vi "meter_buffered - one channel.vi"(7 "Samples":dbl=50.0 format="%#_13g", 8 "error in":errorcluster, 9 "Channel":u16(ring) items=["PD 1", "PD 2", "PD 3"], 10 "PD Range":dbl=3e-05 format="%#_13g", 11 "meter-VISA":refnum<visa-resource-name>) -> (0 "error out":errorcluster, 1 "avg":dbl, 2 "ch data":dbl[](array[numeric]), 3 "meter-VISA-out":refnum<visa-resource-name>, 4 "stdev":dbl)   [LabVIEW 2024]
uses:
  <instrlib>/Keithley 6517/Keithley 6517.lvlib
  <vilib>/Analysis/NI_AALBase.lvlib
panel:
  out "read buffer":string
  out "vi_runtime":u32
  out "pd1_size":i32
  out "pd1_data":dbl[](array[numeric])
  out "cmd":string
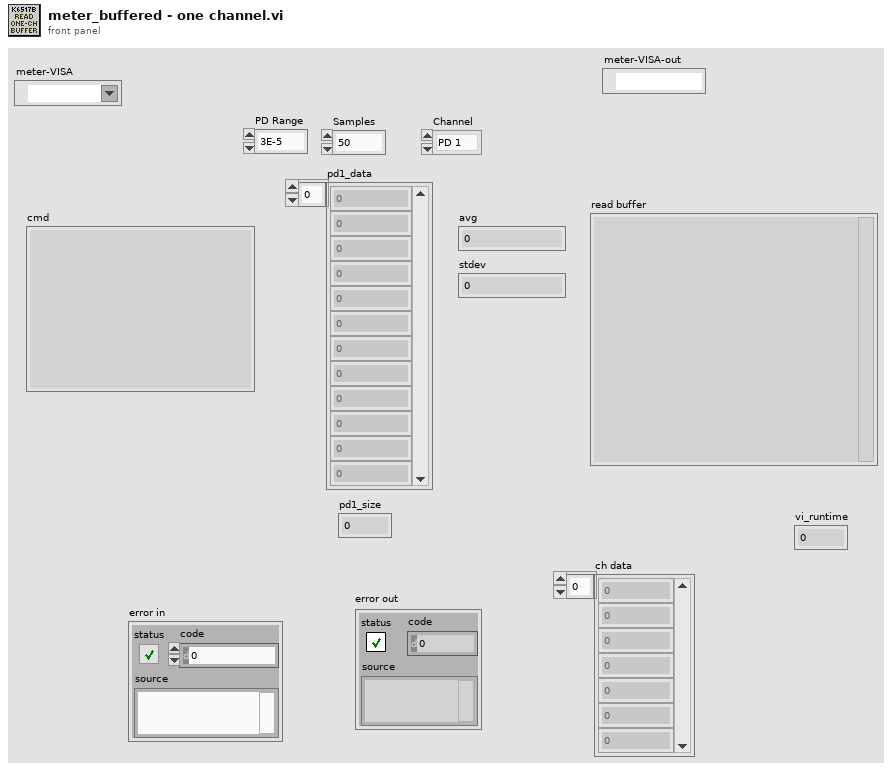
[diagram p1: front panel]
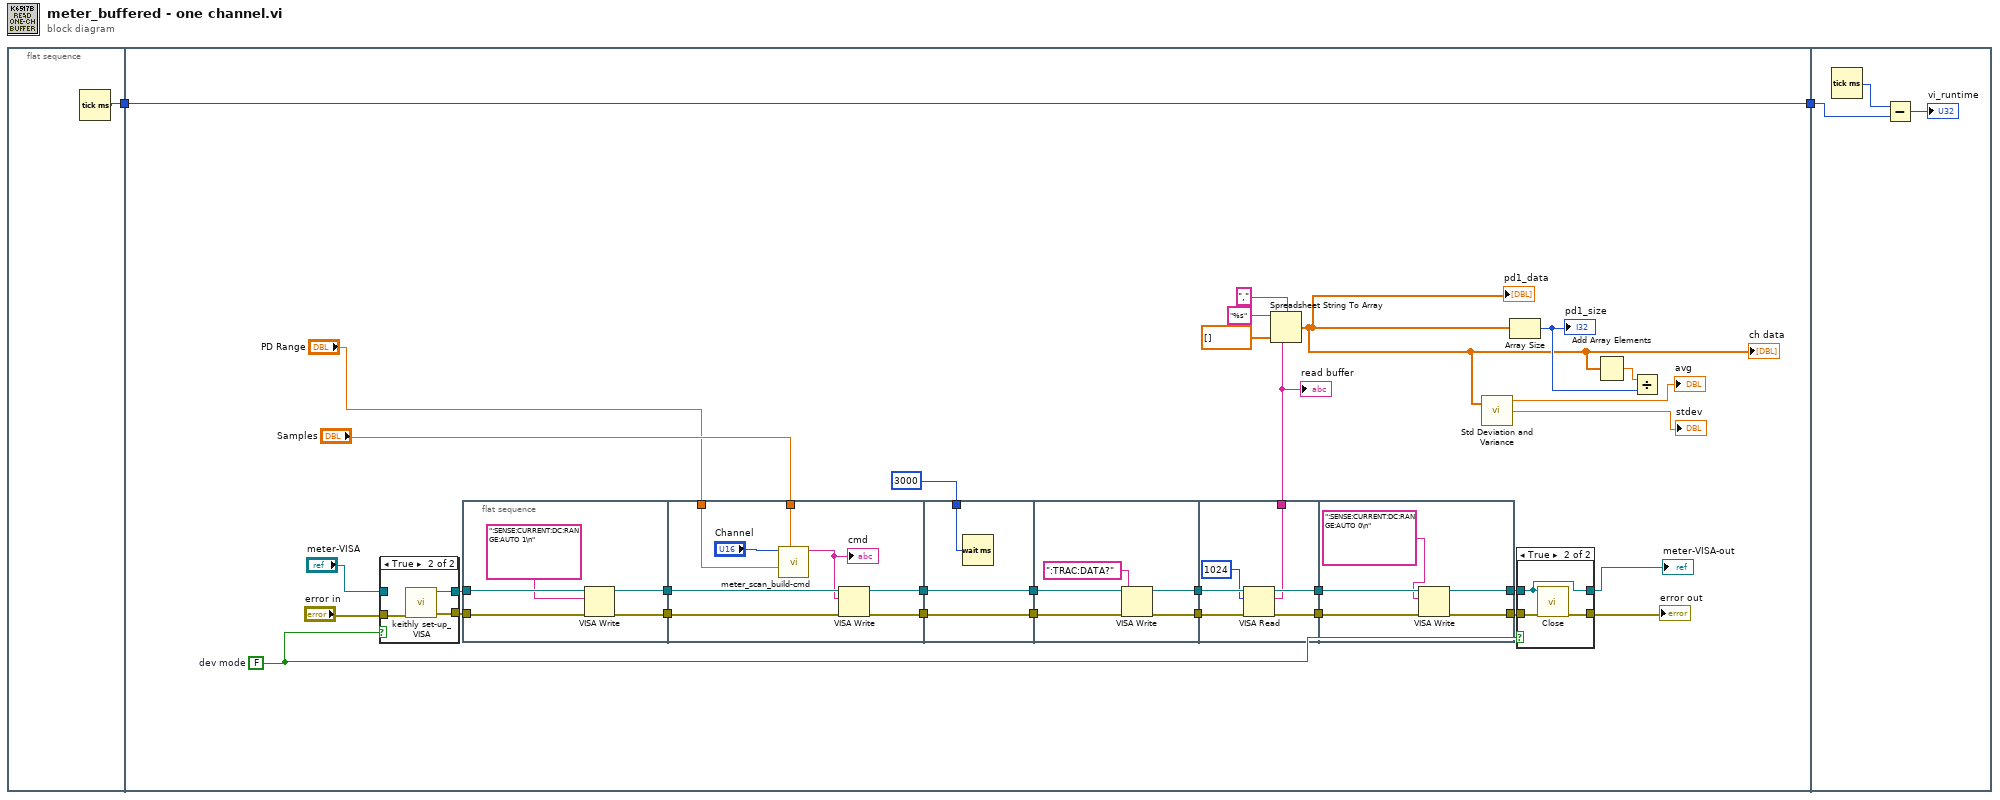
[diagram p0: block diagram]
diagram:
  n1 = flat-sequence {
    tunnel: [w3] -> w1
    tunnel: [w16] -> w2
    tunnel: w1 -> [w16]
    tunnel: w2 -> [w79]
    frame #0 {
      n2 = Tick Count (ms)() -> (millisecond timer value=w3:u32)
    }
    frame #1 {
      w24 = FALSE  # dev mode
      n3 = case shown="True" w24 {
        tunnel: "error in" -> [w73 w77]
        tunnel: [w74 w76] -> w27
        tunnel: [w73 w75] -> w26
        tunnel: "meter-VISA" -> [w74 _]
        frame False {
        }
        frame True {
          n4 = call "keithly set-up_VISA.vi"("error in"=w77) -> ("error out"=w75:errorcluster, "meter-VISA"=w76:refnum<visa-resource-name>)  [unwired: 9 in]
        }
      }
      n5 = flat-sequence {
        tunnel: w26 -> [w38]
        tunnel: w27 -> [w40]
        tunnel: [w39] -> w10
        tunnel: [w37] -> w9
        tunnel: [w46] -> w35
        tunnel: [w45] -> w34
        tunnel: "Samples" -> [w43]
        tunnel: "PD Range" -> [w41]
        tunnel: w10 -> [w48]
        tunnel: w9 -> [w47]
        tunnel: w35 -> [w51]
        tunnel: [w51] -> w33
        tunnel: w34 -> [w50]
        tunnel: [w50] -> w32
        tunnel: u32 3000 ("milliseconds to wait") -> [w49]
        tunnel: [w53] -> w31
        tunnel: [w52] -> w30
        tunnel: w33 -> [w56]
        tunnel: w32 -> [w54]
        tunnel: w31 -> [w62]
        tunnel: w30 -> [w61]
        tunnel: [w58] -> w22
        tunnel: [w60] -> w8
        tunnel: [w59] -> w7
        tunnel: [w65] -> w14
        tunnel: [w64] -> w13
        tunnel: w8 -> [w67]
        tunnel: w7 -> [w66]
        frame #0 {
          n6 = VISA Write(VISA resource name=w40, write buffer=":SENSE:CURRENT:DC:RANGE:AUTO 1\n", error in (no error)=w38) -> (VISA resource name out=w39:refnum<visa-resource-name>, error out=w37:errorcluster)  [unwired: 1 out]
        }
        frame #1 {
          n7 = call "meter_scan_build-cmd.vi"("Samples"=w43, "Range"=w41, "Channel"="Channel") -> ("Command"=w42:string)  [unwired: 8 in]
          "cmd" <- w42
          n8 = VISA Write(VISA resource name=w48, write buffer=w42, error in (no error)=w47) -> (VISA resource name out=w45:refnum<visa-resource-name>, error out=w46:errorcluster)  [unwired: 1 out]
        }
        frame #2 {
          n9 = Wait (ms)(milliseconds to wait=w49) -> ()  [unwired: 1 out]
        }
        frame #3 {
          n10 = VISA Write(VISA resource name=w54, write buffer=":TRAC:DATA?" ("String"), error in (no error)=w56) -> (VISA resource name out=w52:refnum<visa-resource-name>, error out=w53:errorcluster)  [unwired: 1 out]
        }
        frame #4 {
          n11 = VISA Read(VISA resource name=w61, byte count=u32 1024, error in (no error)=w62) -> (VISA resource name out=w59:refnum<visa-resource-name>, read buffer=w58:string, error out=w60:errorcluster)  [unwired: 1 out]
        }
        frame #5 {
          n12 = VISA Write(VISA resource name=w66, write buffer=":SENSE:CURRENT:DC:RANGE:AUTO 0\n", error in (no error)=w67) -> (VISA resource name out=w65:refnum<visa-resource-name>, error out=w64:errorcluster)  [unwired: 1 out]
        }
      }
      n13 = Spreadsheet String To Array(delimiter (Tab)=",", format string="%s", spreadsheet string=w22, array type (2D Dbl)=dbl[] []) -> (array=w6:dbl[])
      "pd1_data" <- w6
      "ch data" <- w6
      n14 = call <vilib>:"Std Deviation and Variance.vi"("X"=w6) -> ("mean"=→"avg":dbl, "standard deviation"=→"stdev":dbl)  [unwired: 1 in, 1 out]
      n15 = Array Size(array=w6) -> (size(s)=w11:i32)
      "pd1_size" <- w11
      n16 = case shown="True" w24 {
        tunnel: [w69 w72] -> w29
        tunnel: w13 -> [w69 w71]
        tunnel: w14 -> [w68 w70]
        tunnel: [w68 w70] -> w23
        frame False {
        }
        frame True {
          n17 = call <instrlib>:"Close.vi"("error in (no error)"=w71, "VISA resource name"=w70) -> ("error out"=w72:errorcluster)  [unwired: 9 in]
        }
      }
      "error out" <- w29
      "meter-VISA-out" <- w23
      n18 = Add Array Elements(numeric array=w6) -> (sum=w12:dbl)
      n19 = Divide(x=w12, y=w11) -> ()  [unwired: 1 out]
      "read buffer" <- w22
    }
    frame #2 {
      n20 = Tick Count (ms)() -> (millisecond timer value=w80:u32)
      n21 = Subtract(x=w80, y=w79) -> (x-y=→"vi_runtime":u32)
    }
  }
